vi "env-toolkit.vi"() -> (0 "error out":errorcluster)   [LabVIEW 2025]
doc: "Environment Toolkit for TestStand - Command Line Interface"
uses:
  Type Definitions/CLI State--enum.ctl
  Type Definitions/CLI Data--cluster.ctl
  ITSDiscovery/ITSDiscovery.lvclass
  IProcess Executor/IProcess Executor.lvclass
  Type Definitions/Architecture--enum.ctl
  Process Executor/Process Executor.lvclass
  TSDiscovery/TSDiscovery.lvclass
  Type Definitions/Profile--cluster.ctl
  Type Definitions/Execution Plan--cluster.ctl
  <vilib>/Utility/error.llb/DialogType.ctl
  <vilib>/Wiresmith Technology/G CLI/CLI Class/CLI.lvclass
  Libraries/TS Environment Manager/TS Environment Manager.lvlib
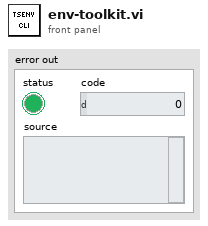
[diagram p1: front panel]
types:
  T1 = typedef "CLI Data--cluster.ctl" = cluster{"Name":string, "Architecture":T2, "File":path, "Command":string, "ITSDiscovery.lvclass":refnum<class "ITSDiscovery.lvclass">, "IProcess Executor.lvclass":refnum<class "IProcess Executor.lvclass">, "Version":string, "Message":string}
  T2 = typedef "Architecture--enum.ctl" = enum16{"32bit", "64bit"}
  T3 = typedef "CLI State--enum.ctl" = enum16{"Init", "Run", "Error", "Exit"}
  T4 = typedef "Profile--cluster.ctl" = cluster{"Name":string, "Version":string, "Architecture":T2, "Environment":path}
  T5 = typedef "Execution Plan--cluster.ctl" = cluster{"Exe Path":path, "Args":string[], "Timeout":i32}
  T6 = typedef "TSInstall--cluster.ctl" = cluster{"Version":string, "Architecture":T2, "Version Key":string, "ID":string}
  T7 = typedef "DialogType.ctl" = u16
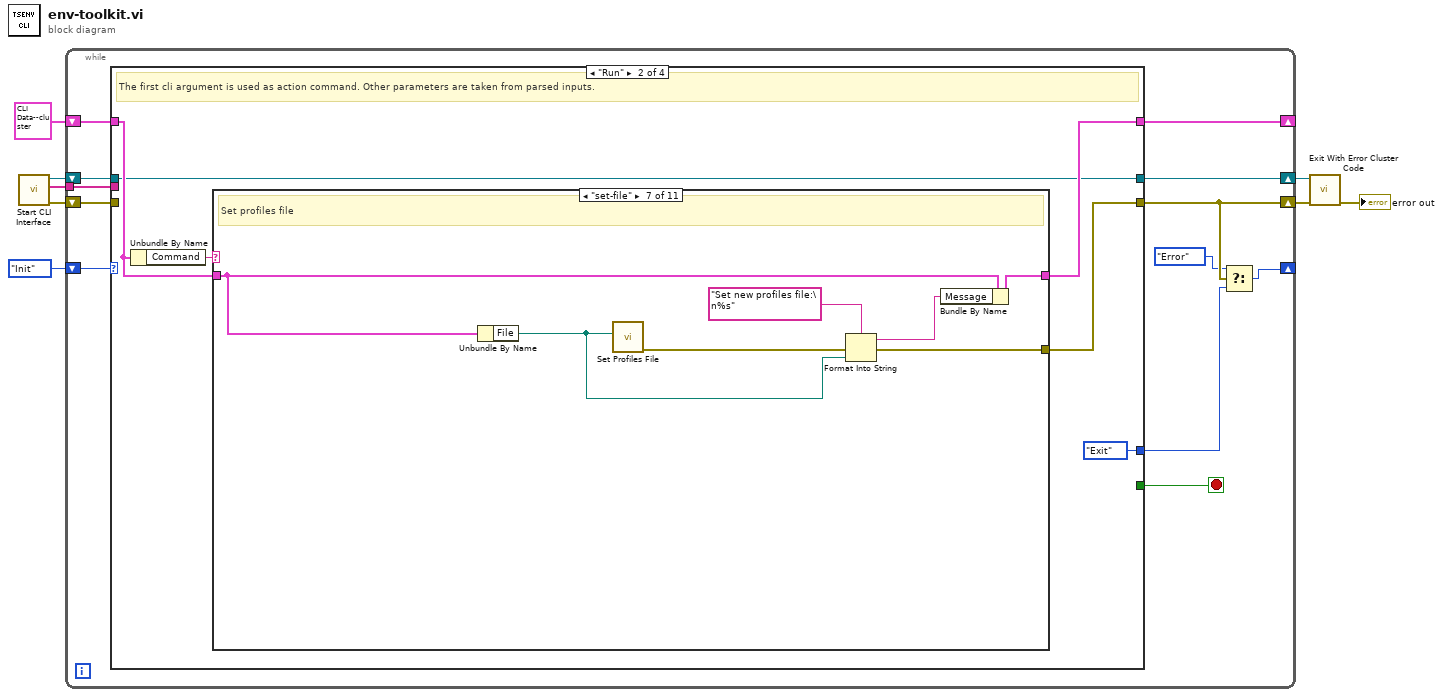
[diagram p0: block diagram]
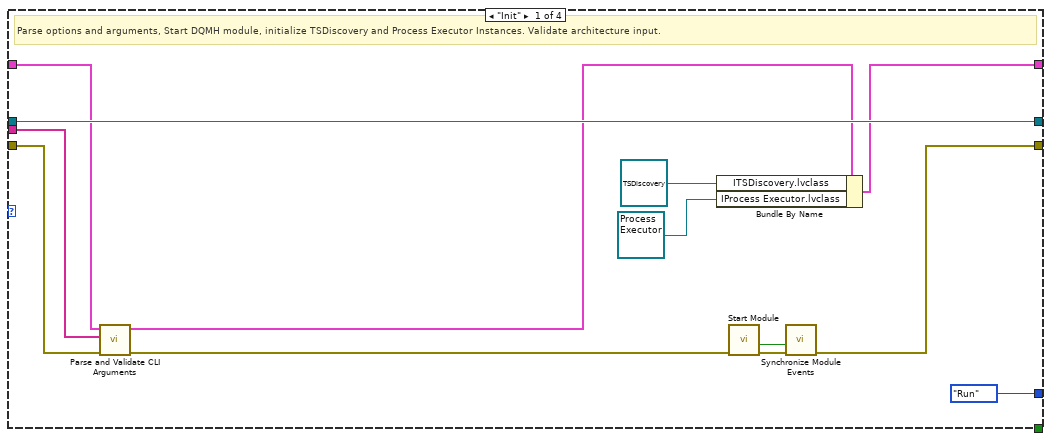
[diagram p2: hidden frame]
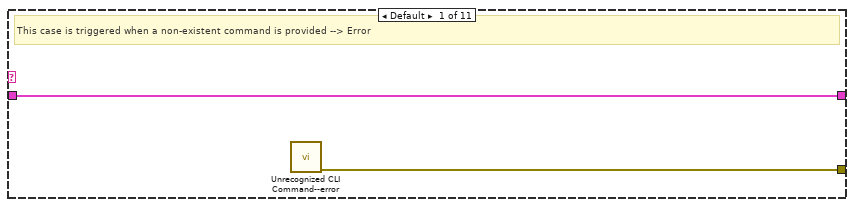
[diagram p3: hidden frame]
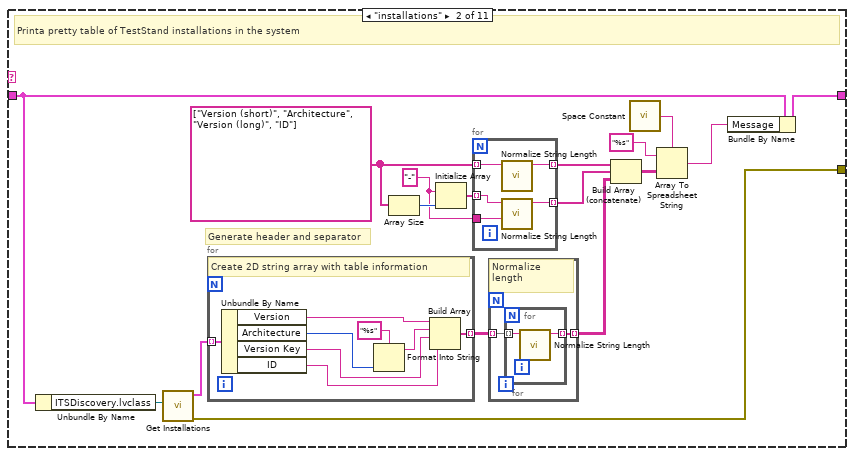
[diagram p4: hidden frame]
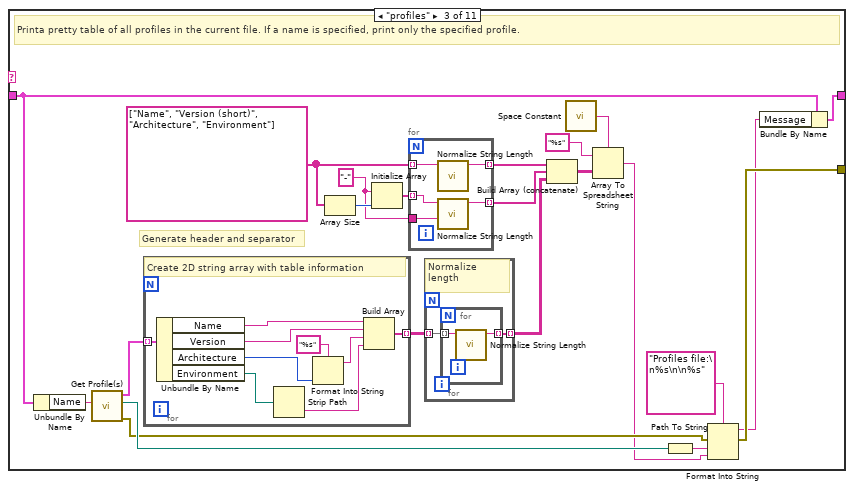
[diagram p5: hidden frame]
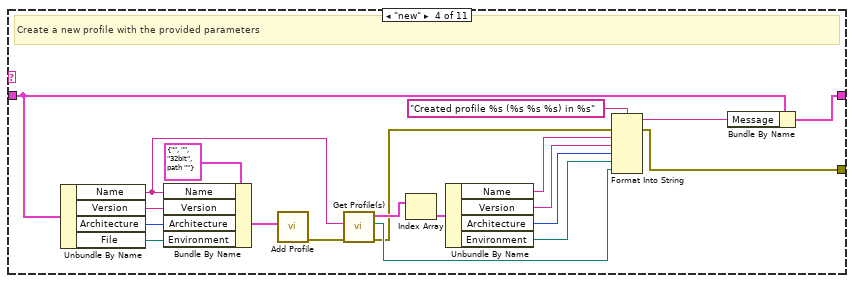
[diagram p6: hidden frame]
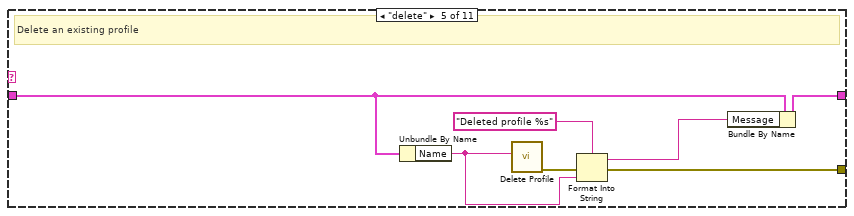
[diagram p7: hidden frame]
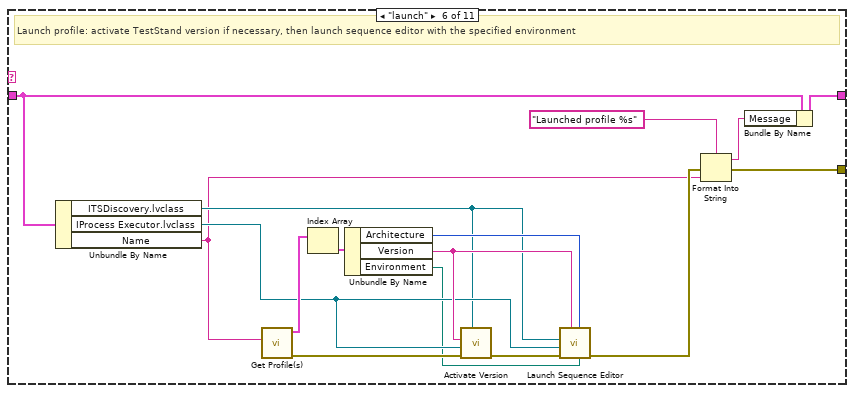
[diagram p8: hidden frame]
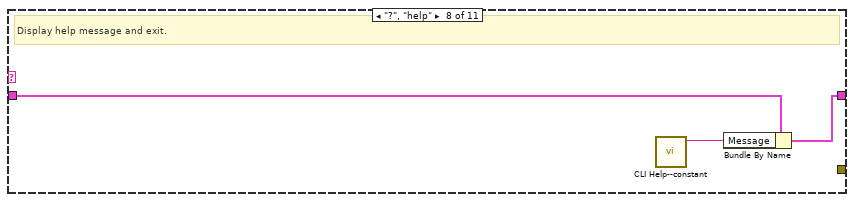
[diagram p9: hidden frame]
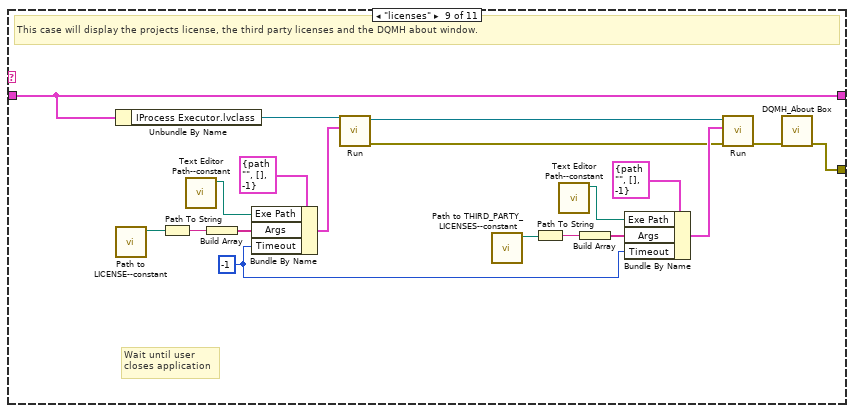
[diagram p10: hidden frame]
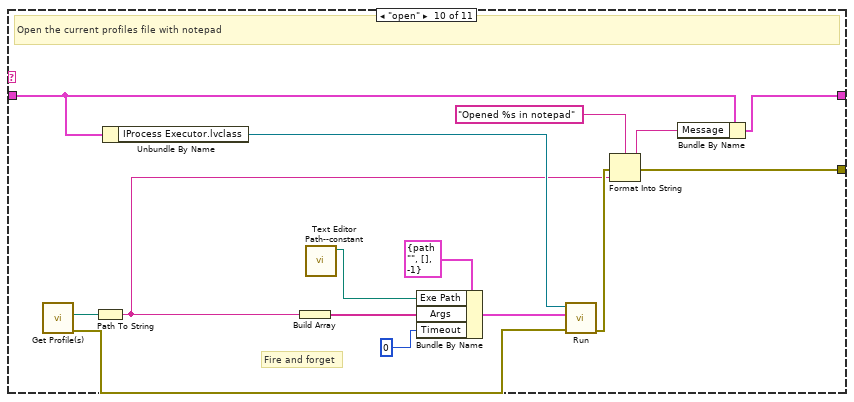
[diagram p11: hidden frame]
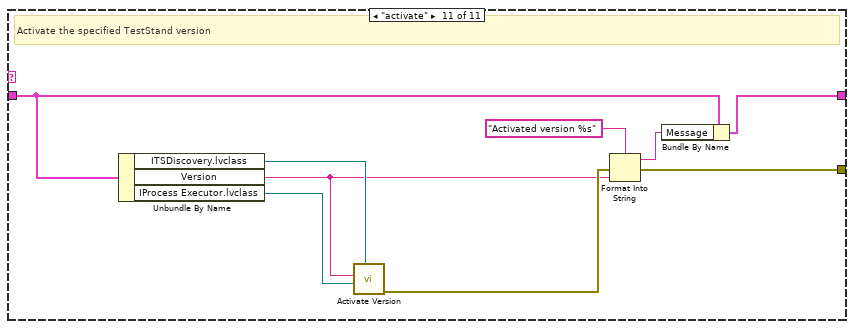
[diagram p12: hidden frame]
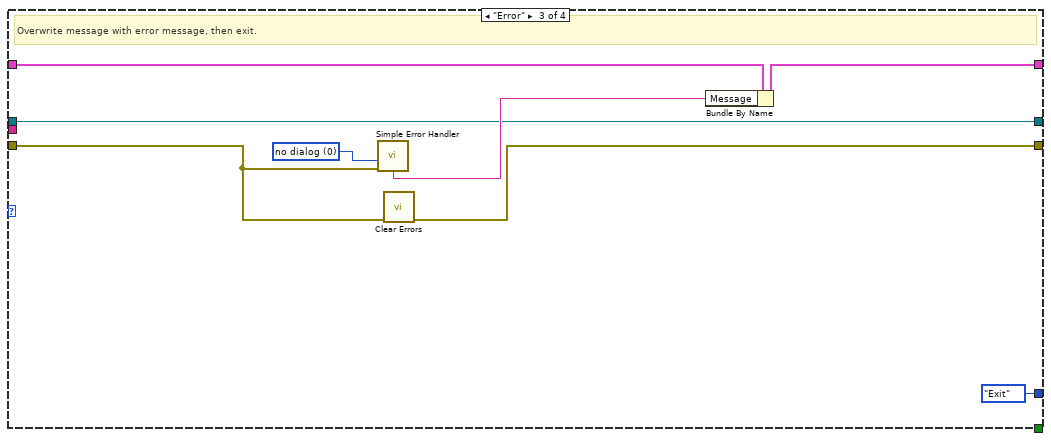
[diagram p13: hidden frame]
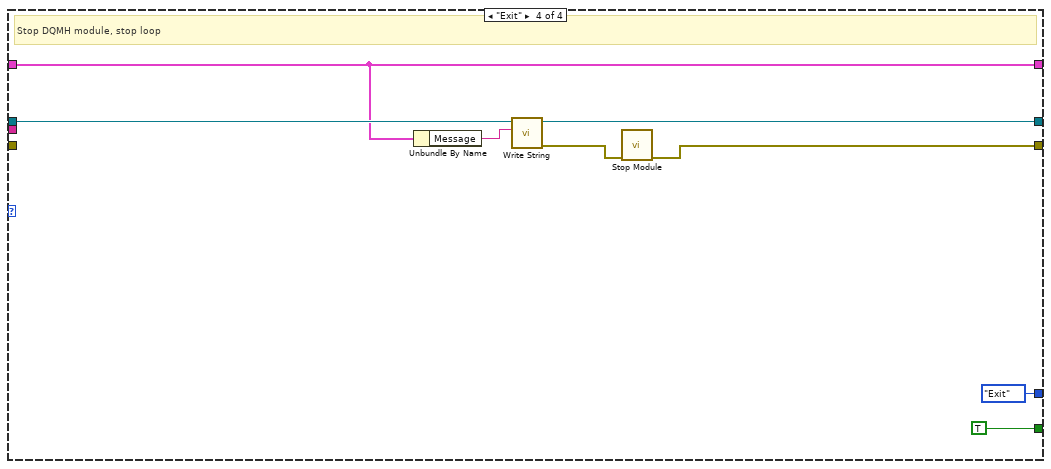
[diagram p14: hidden frame]
diagram:
  n1 = call <vilib>:"Start CLI Interface.vi"() -> ("error out"=w6:errorcluster, "Custom Parameters"=w5:string[], "CLI out"=w7:refnum<class "CLI.lvclass">)  [unwired: 8 in, 1 out]
  n2 = while {
    shift-right: [w16] -> _
    shift-left: CLI_State--enum."Init" -> [w20]
    shift-right: [w18] -> w4
    shift-left: w6 -> [w10]
    tunnel: w5 -> [w15]
    shift-right: [w13] -> w3
    shift-left: w7 -> [w14]
    shift-right: [w11] -> _
    shift-left: T1 {"Name"="", "Architecture"=enum."32bit", "File"=path "", "Command"="", "ITSDiscovery.lvclass"=refnum, "IProcess Executor.lvclass"=refnum, "Version"="", "Message"=""} ("CLI Data") -> [w12]
    stop <- w19 stop-if-true
    n3 = case shown="\"Run\"" w20 {
      tunnel: [_ _ _ TRUE] -> w19
      tunnel: [w21 w38 w212 w226] -> w18
      tunnel: w15 -> [w29 _ _ _]
      tunnel: w14 -> [w33 w34 w213 w223]
      tunnel: [w33 w34 w213 w224] -> w13
      tunnel: w12 -> [w32 w36 w214 w221]
      tunnel: [w24 w35 w215 w221] -> w11
      tunnel: w10 -> [w31 _ w219 _]
      tunnel: [CLI_State--enum."Run" CLI_State--enum."Exit" CLI_State--enum."Exit" CLI_State--enum."Exit"] -> w9
      frame "Init" {
        # "Parse options and arguments, Start DQMH module, initialize TSDiscovery and Process Executor Instances. Validate architecture input."
        n4 = call "Parse and Validate CLI Arguments.vi"("error in"=w31, "Custom Parameters"=w29, "CLI Data in"=w32) -> ("error out"=w26:errorcluster, "CLI Data out"=w25:T1)  [unwired: 7 in]
        n5 = Bundle By Name(cluster=w25, "ITSDiscovery.lvclass"=refnum<class "TSDiscovery.lvclass"> refnum ("TSDiscovery.lvclass"), "IProcess Executor.lvclass"=refnum<class "Process Executor.lvclass"> refnum ("Process Executor.lvclass")) -> (w24:T1)
        n6 = call "Start Module.vi"("error in"=w26) -> ("error out"=w28:errorcluster, "Wait for Event Sync?"=w27:bool)  [unwired: 6 in, 3 out]
        n7 = call "Synchronize Module Events.vi"("error in"=w28, "Wait for Event Sync?"=w27) -> ("error out"=w21:errorcluster)  [unwired: 9 in]
      }
      frame "Run" {
        # "The first cli argument is used as action command. Other parameters are taken from parsed inputs."
        n8 = Unbundle By Name(w36) -> ("Command"=w39:string)
        n9 = case shown="\"set-file\"" w39 {
          tunnel: [w41 w45 w78 w117 w138 w146 w161 _ w187 w191 w205] -> w38
          tunnel: w36 -> [w40 w44 w80 w120 w141 w150 w165 w168 w176 w194 w208]
          tunnel: [w40 w42 w79 w118 w139 w149 w164 w167 w176 w195 w209] -> w35
          frame Default {
            # "This case is triggered when a non-existent command is provided --> Error"
            n10 = call "Unrecognized CLI Command--error.vi"() -> ("error out"=w41:errorcluster)  [unwired: 11 in]
          }
          frame "installations" {
            w54 = "-"
            w57 = string[] ["Version (short)", "Architecture", "Version (long)", "ID"]
            # "Generate header and separator"
            # "Printa pretty table of TestStand installations in the system"
            n11 = Unbundle By Name(w44) -> ("ITSDiscovery.lvclass"=w58:refnum<class "ITSDiscovery.lvclass">)
            n12 = call "Get Installations.vi"("ITSDiscovery.lvclass"=w58) -> ("error out"=w45:errorcluster, "Installations"=w53:T6[])  [unwired: 8 in, 1 out]
            n13 = for {
              tunnel: w53 -> [w70] mode=indexing
              tunnel: [w63] -> w52 mode=indexing
              # "Create 2D string array with table information"
              n14 = Unbundle By Name(w70) -> ("Version"=w67:string, "Architecture"=w68:T2, "Version Key"=w65:string, "ID"=w64:string)
              n15 = Format Into String(format string="%s", w68) -> (resulting string=w66:string)  [unwired: 2 in, 1 out]
              n16 = Build Array(w67, w66, w65, w64) -> (w63:string[])
            }
            n17 = Array Size(array=w57) -> (size(s)=w56:i32)
            n18 = Initialize Array(w54, w56) -> (w55:string[])
            n19 = for {
              tunnel: w57 -> [w75] mode=indexing
              tunnel: w55 -> [w74] mode=indexing
              tunnel: w54 -> [w73]
              tunnel: [w72] -> w51 mode=indexing
              tunnel: [w71] -> w50 mode=indexing
              n20 = call "Normalize String Length.vi"("String in"=w75) -> ("Normalized String"=w72:string)  [unwired: 10 in]
              n21 = call "Normalize String Length.vi"("Fill with"=w73, "String in"=w74) -> ("Normalized String"=w71:string)  [unwired: 9 in]
            }
            n22 = for {
              tunnel: w52 -> [w60] mode=indexing
              tunnel: [w59] -> w49 mode=indexing
              # "Normalize length"
              n23 = for {
                tunnel: w60 -> [w62] mode=indexing
                tunnel: [w61] -> w59 mode=indexing
                n24 = call "Normalize String Length.vi"("String in"=w62) -> ("Normalized String"=w61:string)  [unwired: 10 in]
              }
            }
            n25 = Build Array (concatenate)(w51, w50, w49) -> (w48:string[][])
            n26 = call <vilib>:"Space Constant.vi"() -> ("String"=w47:string)
            n27 = Array To Spreadsheet String(delimiter (Tab)=w47, array=w48, 3:"%s" ("format string")) -> (spreadsheet string=w43:string)
            n28 = Bundle By Name(cluster=w44, "Message"=w43) -> (w42:T1)
          }
          frame "profiles" {
            w94 = "-"
            w97 = string[] ["Name", "Version (short)", "Architecture", "Environment"]
            # "Generate header and separator"
            # "Printa pretty table of all profiles in the current file. If a name is specified, print only the specified profile."
            n29 = Unbundle By Name(w80) -> ("Name"=w86:string)
            n30 = call "Get Profile(s).vi"("Name"=w86) -> ("error out"=w81:errorcluster, "File"=w83:path, "Profile(s)"=w85:T4[])  [unwired: 7 in, 1 out]
            n31 = for {
              tunnel: w85 -> [w110] mode=indexing
              tunnel: [w107] -> w93 mode=indexing
              # "Create 2D string array with table information"
              n32 = Unbundle By Name(w110) -> ("Name"=w108:string, "Version"=w104:string, "Architecture"=w106:T2, "Environment"=w103:path)
              n33 = Strip Path(path=w103) -> (name=w102:string)  [unwired: 1 out]
              n34 = Format Into String(format string="%s", w106) -> (resulting string=w105:string)  [unwired: 2 in, 1 out]
              n35 = Build Array(w108, w104, w105, w102) -> (w107:string[])
            }
            n36 = Array Size(array=w97) -> (size(s)=w96:i32)
            n37 = Initialize Array(w94, w96) -> (w95:string[])
            n38 = for {
              tunnel: w97 -> [w115] mode=indexing
              tunnel: w95 -> [w114] mode=indexing
              tunnel: w94 -> [w113]
              tunnel: [w112] -> w92 mode=indexing
              tunnel: [w111] -> w91 mode=indexing
              n39 = call "Normalize String Length.vi"("String in"=w115) -> ("Normalized String"=w112:string)  [unwired: 10 in]
              n40 = call "Normalize String Length.vi"("Fill with"=w113, "String in"=w114) -> ("Normalized String"=w111:string)  [unwired: 9 in]
            }
            n41 = for {
              tunnel: w93 -> [w99] mode=indexing
              tunnel: [w98] -> w90 mode=indexing
              # "Normalize length"
              n42 = for {
                tunnel: w99 -> [w101] mode=indexing
                tunnel: [w100] -> w98 mode=indexing
                n43 = call "Normalize String Length.vi"("String in"=w101) -> ("Normalized String"=w100:string)  [unwired: 10 in]
              }
            }
            n44 = Build Array (concatenate)(w92, w91, w90) -> (w89:string[][])
            n45 = call <vilib>:"Space Constant.vi"() -> ("String"=w88:string)
            n46 = Array To Spreadsheet String(delimiter (Tab)=w88, array=w89, 3:"%s" ("format string")) -> (spreadsheet string=w77:string)
            n47 = Path To String(path=w83) -> (string=w82:string)
            n48 = Format Into String(format string="Profiles file:\n%s\n\n%s", error in=w81, w82, w77) -> (resulting string=w76:string, error out=w78:errorcluster)  [unwired: 1 in]
            n49 = Bundle By Name(cluster=w80, "Message"=w76) -> (w79:T1)
          }
          frame "new" {
            # "Create a new profile with the provided parameters"
            n50 = Unbundle By Name(w120) -> ("Name"=w130:string, "Version"=w134:string, "Architecture"=w133:T2, "File"=w132:path)
            n51 = Bundle By Name(cluster=T4 {"Name"="", "Version"="", "Architecture"=enum."32bit", "Environment"=path ""} ("Profile"), "Name"=w130, "Version"=w134, "Architecture"=w133, "Environment"=w132) -> (w116:T4)
            n52 = call "Add Profile.vi"("Profile"=w116) -> ("error out"=w131:errorcluster)  [unwired: 9 in, 1 out]
            n53 = call "Get Profile(s).vi"("error in"=w131, "Name"=w130) -> ("error out"=w121:errorcluster, "File"=w122:path, "Profile(s)"=w129:T4[])  [unwired: 6 in, 1 out]
            n54 = Index Array(array=w129) -> (element=w128:T4)  [unwired: 1 in]
            n55 = Unbundle By Name(w128) -> ("Name"=w126:string, "Version"=w125:string, "Architecture"=w124:T2, "Environment"=w123:path)
            n56 = Format Into String(format string="Created profile %s (%s %s %s) in %s", error in=w121, w126, w125, w124, w123, w122) -> (resulting string=w119:string, error out=w117:errorcluster)  [unwired: 1 in]
            n57 = Bundle By Name(cluster=w120, "Message"=w119) -> (w118:T1)
          }
          frame "delete" {
            # "Delete an existing profile"
            n58 = Unbundle By Name(w141) -> ("Name"=w136:string)
            n59 = call "Delete Profile.vi"("Name"=w136) -> ("error out"=w137:errorcluster)  [unwired: 9 in, 1 out]
            n60 = Format Into String(format string="Deleted profile %s", error in=w137, w136) -> (resulting string=w140:string, error out=w138:errorcluster)  [unwired: 1 in]
            n61 = Bundle By Name(cluster=w141, "Message"=w140) -> (w139:T1)
          }
          frame "launch" {
            # "Launch profile: activate TestStand version if necessary, then launch sequence editor with the specified environment"
            n62 = Unbundle By Name(w150) -> ("ITSDiscovery.lvclass"=w151:refnum<class "ITSDiscovery.lvclass">, "IProcess Executor.lvclass"=w152:refnum<class "IProcess Executor.lvclass">, "Name"=w145:string)
            n63 = call "Get Profile(s).vi"("Name"=w145) -> ("error out"=w156:errorcluster, "Profile(s)"=w158:T4[])  [unwired: 7 in, 2 out]
            n64 = Index Array(array=w158) -> (element=w157:T4)  [unwired: 1 in]
            n65 = Unbundle By Name(w157) -> ("Architecture"=w153:T2, "Version"=w154:string, "Environment"=w143:path)
            n66 = call "Activate Version.vi"("ITSDiscovery.lvclass"=w151, "error in"=w156, "IProcess Executor.lvclass"=w152, "Version"=w154) -> ("error out"=w155:errorcluster)  [unwired: 6 in, 1 out]
            n67 = call "Launch Sequence Editor.vi"("Environment"=w143, "Architecture"=w153, "Version"=w154, "error in"=w155, "IProcess Executor.lvclass"=w152, "ITSDiscovery.lvclass"=w151) -> ("error out"=w147:errorcluster)  [unwired: 4 in, 1 out]
            n68 = Format Into String(format string="Launched profile %s", error in=w147, w145) -> (resulting string=w144:string, error out=w146:errorcluster)  [unwired: 1 in]
            n69 = Bundle By Name(cluster=w150, "Message"=w144) -> (w149:T1)
          }
          frame "set-file" {
            # "Set profiles file"
            n70 = Unbundle By Name(w165) -> ("File"=w160:path)
            n71 = call "Set Profiles File.vi"("File Path"=w160) -> ("error out"=w162:errorcluster)  [unwired: 9 in, 1 out]
            n72 = Format Into String(format string="Set new profiles file:\n%s", error in=w162, w160) -> (resulting string=w159:string, error out=w161:errorcluster)  [unwired: 1 in]
            n73 = Bundle By Name(cluster=w165, "Message"=w159) -> (w164:T1)
          }
          frame "?", "help" {
            # "Display help message and exit."
            n74 = call "CLI Help--constant.vi"() -> ("Help Message"=w166:string)  [unwired: 11 in]
            n75 = Bundle By Name(cluster=w168, "Message"=w166) -> (w167:T1)
          }
          frame "licenses" {
            w178 = -1 ("Timeout")
            # "Wait until user\ncloses application"
            # "This case will display the projects license, the third party licenses and the DQMH about window."
            n76 = Unbundle By Name(w176) -> ("IProcess Executor.lvclass"=w175:refnum<class "IProcess Executor.lvclass">)
            n77 = call "Path to LICENSE--constant.vi"() -> ("appended path"=w177:path)  [unwired: 11 in]
            n78 = Path To String(path=w177) -> (string=w184:string)
            n79 = call "Text Editor Path--constant.vi"() -> ("Path"=w183:path)  [unwired: 11 in]
            n80 = Build Array(w184) -> (w185:string[])
            n81 = Bundle By Name(cluster=T5 {"Exe Path"=path "", "Args"=[], "Timeout"=-1} ("Execution Plan"), "Exe Path"=w183, "Args"=w185, "Timeout"=w178) -> (w174:T5)
            n82 = call-dynamic "Run.vi"("Execution Plan"=w174, "IProcess Executor in"=w175) -> ("error out"=w171:errorcluster, "IProcess Executor out"=w173:refnum<class "IProcess Executor.lvclass">)  [unwired: 8 in]
            n83 = call "Path to THIRD_PARTY_LICENSES--constant.vi"() -> ("appended path"=w169:path)  [unwired: 11 in]
            n84 = Path To String(path=w169) -> (string=w180:string)
            n85 = call "Text Editor Path--constant.vi"() -> ("Path"=w179:path)  [unwired: 11 in]
            n86 = Build Array(w180) -> (w181:string[])
            n87 = Bundle By Name(cluster=T5 {"Exe Path"=path "", "Args"=[], "Timeout"=-1} ("Execution Plan"), "Exe Path"=w179, "Args"=w181, "Timeout"=w178) -> (w172:T5)
            n88 = call-dynamic "Run.vi"("error in"=w171, "Execution Plan"=w172, "IProcess Executor in"=w173) -> ("error out"=w170:errorcluster)  [unwired: 7 in, 1 out]
            n89 = call <vilib>:"DQMH_About Box.vi"("error in"=w170) -> ("error out"=w187:errorcluster)  [unwired: 10 in]
          }
          frame "open" {
            # "Fire and forget"
            # "Open the current profiles file with notepad"
            n90 = call "Get Profile(s).vi"() -> ("error out"=w196:errorcluster, "File"=w202:path)  [unwired: 8 in, 2 out]
            n91 = Path To String(path=w202) -> (string=w190:string)
            n92 = Unbundle By Name(w194) -> ("IProcess Executor.lvclass"=w198:refnum<class "IProcess Executor.lvclass">)
            n93 = Build Array(w190) -> (w200:string[])
            n94 = call "Text Editor Path--constant.vi"() -> ("Path"=w188:path)  [unwired: 11 in]
            n95 = Bundle By Name(cluster=T5 {"Exe Path"=path "", "Args"=[], "Timeout"=-1} ("Execution Plan"), "Exe Path"=w188, "Args"=w200, "Timeout"=0) -> (w197:T5)
            n96 = call-dynamic "Run.vi"("error in"=w196, "Execution Plan"=w197, "IProcess Executor in"=w198) -> ("error out"=w192:errorcluster)  [unwired: 7 in, 1 out]
            n97 = Format Into String(format string="Opened %s in notepad", error in=w192, w190) -> (resulting string=w189:string, error out=w191:errorcluster)  [unwired: 1 in]
            n98 = Bundle By Name(cluster=w194, "Message"=w189) -> (w195:T1)
          }
          frame "activate" {
            # "Activate the specified TestStand version"
            n99 = Unbundle By Name(w208) -> ("ITSDiscovery.lvclass"=w210:refnum<class "ITSDiscovery.lvclass">, "Version"=w204:string, "IProcess Executor.lvclass"=w211:refnum<class "IProcess Executor.lvclass">)
            n100 = call "Activate Version.vi"("ITSDiscovery.lvclass"=w210, "IProcess Executor.lvclass"=w211, "Version"=w204) -> ("error out"=w206:errorcluster)  [unwired: 7 in, 1 out]
            n101 = Format Into String(format string="Activated version %s", error in=w206, w204) -> (resulting string=w203:string, error out=w205:errorcluster)  [unwired: 1 in]
            n102 = Bundle By Name(cluster=w208, "Message"=w203) -> (w209:T1)
          }
        }
      }
      frame "Error" {
        w218 = T7 0 items=["no dialog", "OK message", "continue or stop message", "OK message + warnings", "continue/stop + warnings"] ("type of dialog (OK msg:1)")
        # "Overwrite message with error message, then exit."
        n103 = call <vilib>:"Simple Error Handler.vi"("type of dialog (OK msg:1)"=w218, "error in (no error)"=w219) -> ("message"=w216:string)  [unwired: 3 in, 4 out]
        n104 = call <vilib>:"Clear Errors.vi"("error in (no error)"=w219) -> ("error out"=w212:errorcluster)  [unwired: 5 in, 1 out]
        n105 = Bundle By Name(cluster=w214, "Message"=w216) -> (w215:T1)
      }
      frame "Exit" {
        # "Stop DQMH module, stop loop"
        n106 = Unbundle By Name(w221) -> ("Message"=w220:string)
        n107 = call <vilib>:"Write String.vi"("Text to Write"=w220, "CLI in"=w223) -> ("error out"=w222:errorcluster, "CLI out"=w224:refnum<class "CLI.lvclass">)  [unwired: 8 in]
        n108 = call "Stop Module.vi"("error in"=w222) -> ("error out"=w226:errorcluster)  [unwired: 10 in]
      }
    }
    n109 = Select(t=CLI_State--enum."Error", s=w18, f=w9) -> (s? t:f=w16:T3)
  }
  n110 = call <vilib>:"Exit With Error Cluster Code.vi"("error in (no error)"=w4, "CLI in"=w3) -> ("error out"=→"error out":errorcluster)  [unwired: 9 in]
